vi "Get_radius_from_mass.vi"(7 "Density":dbl, 9 "Charge":sgl, 10 "Velocity":sgl, 11 "High Voltage (MV)":sgl) -> (2 "Mass":ext, 3 "Radius":dbl)   [LabVIEW 2012]
panel:
  # "Density of Fe: \n7.874 g·cm-3"
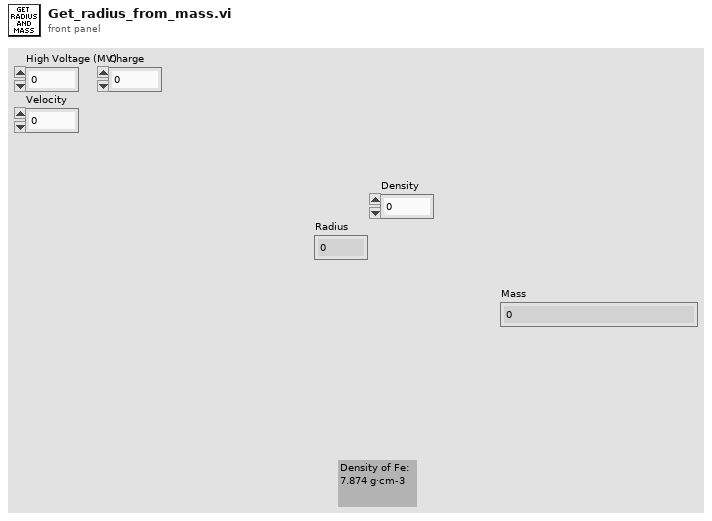
[diagram p1: front panel]
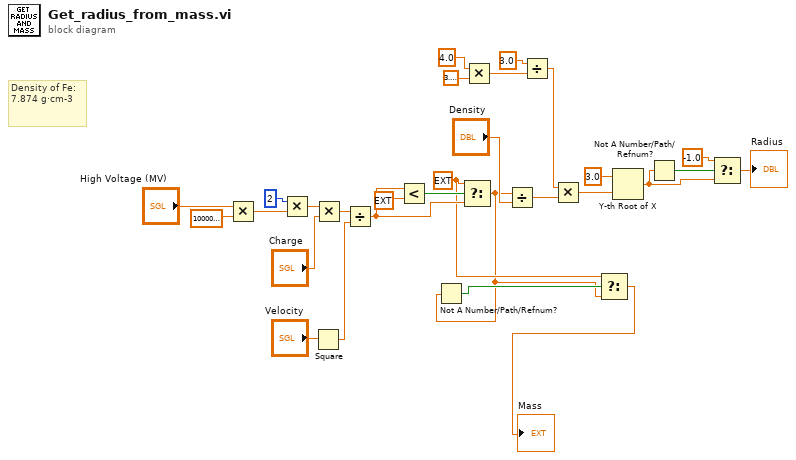
[diagram p0: block diagram]
diagram:
  w4 = ext -1.0 ("y")
  # "Density of Fe: \n7.874 g·cm-3"
  n1 = Multiply(x="High Voltage (MV)", y=sgl 1000000.0) -> (x*y=w7:sgl)
  n2 = Multiply(x=2, y=w7) -> (x*y=w15:sgl)
  n3 = Square(x="Velocity") -> (x^2=w13:sgl)
  n4 = Multiply(x=w15, y="Charge") -> (x*y=w14:sgl)
  n5 = Divide(x=w14, y=w13) -> (x/y=w10:sgl)
  n6 = Less?(x=w10, y=ext 0.0) -> (x < y?=w11:bool)
  n7 = Select(t=w4, s=w11, f=w10) -> (s? t:f=w2:ext)
  n8 = Not A Number/Path/Refnum?(number/path/refnum=w2) -> (NaN/Path/Refnum?=w3:bool)
  n9 = Multiply(x=4.0, y=3.141592653589793) -> (x*y=w26:dbl)
  n10 = Divide(x=w2, y="Density") -> (x/y=w28:ext)
  n11 = Divide(x=3.0, y=w26) -> (x/y=w27:dbl)
  n12 = Multiply(x=w27, y=w28) -> (x*y=w22:ext)
  n13 = Select(t=w4, s=w3, f=w2) -> (s? t:f=→"Mass":ext)
  n14 = Y-th Root of X(1:w22, 2:3.0 ("y")) -> (0:w19:ext)
  n15 = Not A Number/Path/Refnum?(number/path/refnum=w19) -> (NaN/Path/Refnum?=w20:bool)
  n16 = Select(t=-1.0, s=w20, f=w19) -> (s? t:f=→"Radius":ext)
